vi "Get Serial Number.vi"(8 "error in (no error)":errorcluster, 11 "Barcode Reader in":refnum<class "Barcode.lvclass">) -> (0 "error out":errorcluster, 2 "Serial Number":string, 3 "Barcode Reader out":refnum<class "Barcode.lvclass">)   [LabVIEW 2020, in "Barcode Reader Second Iteration.lvlib" / "Barcode.lvclass"]
uses:
  Barcode.lvclass
  Barcode.lvclass/Barcode.ctl
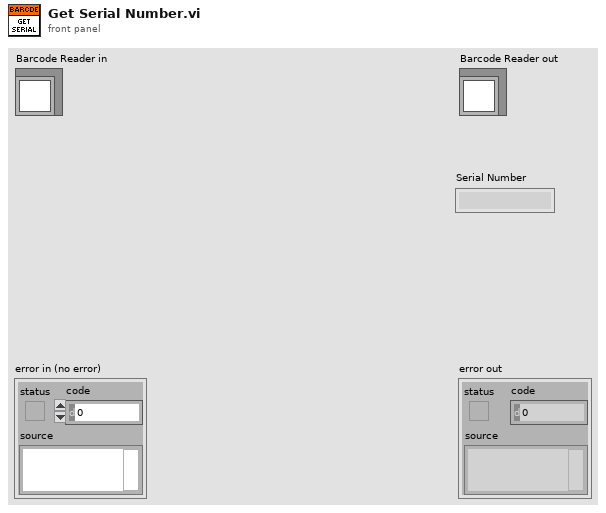
[diagram p1: front panel]
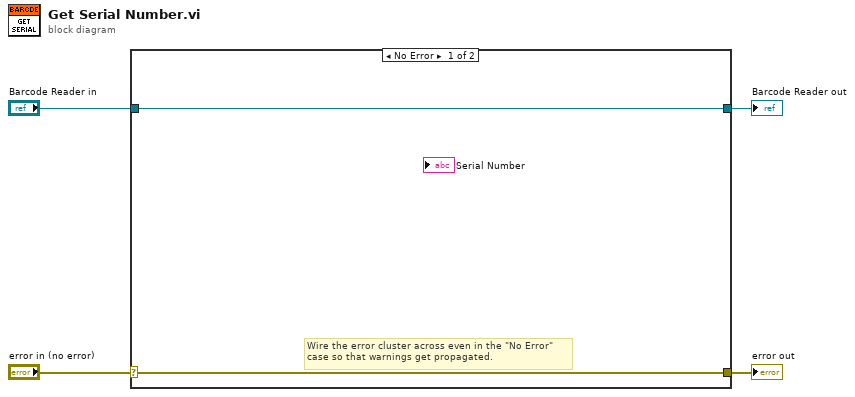
[diagram p0: block diagram]
diagram:
  n1 = case shown="No Error" "error in (no error)" {
    selector: "error in (no error)" -> [w5 w8]
    tunnel: [w5 w8] -> w3
    tunnel: [w6 w7] -> w1
    tunnel: "Barcode Reader in" -> [w6 w7]
    frame No Error {
      # "Wire the error cluster across even in the \"No Error\"\ncase so that warnings get propagated."
    }
    frame Error {
    }
  }
  "error out" <- w3
  "Barcode Reader out" <- w1
